vi "Combine axes arrays.vi"(2 "Axes subset 1":string[](array[string]), 3 "Axes subset 2":string[](array[string])) -> (14 "Combined axes":string[](array[string]), 15 "Double axes":string[](array[string]))   [LabVIEW 2020]
doc: "This VI combines axes from Axes subset 1 and Axes subset 2 and returns the combined and sorted axes array plus axes which had double entries."
panel:
  # "This vi combines axes from Axes subset 1 and Axes subset 2 and returns the \ncombined and sorted axes array plus axes which had double entries."
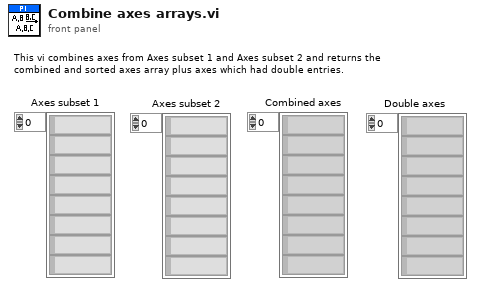
[diagram p1: front panel]
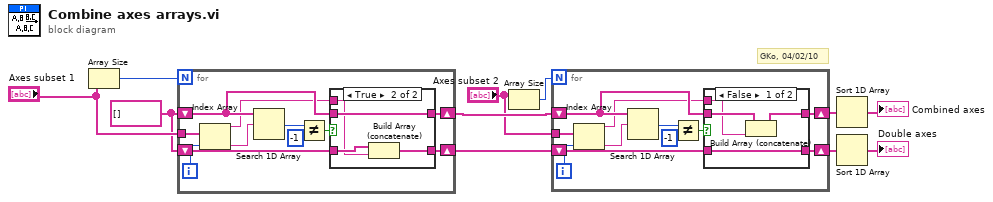
[diagram p0: block diagram]
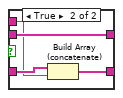
[diagram p2: hidden frame]
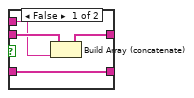
[diagram p3: hidden frame]
diagram:
  w9 = string[] []
  # "GKo, 04/02/10"
  n1 = Array Size(array="Axes subset 1") -> (size(s)=w11:i32)
  n2 = for {
    N: w11 -> [_]
    shift-right: [w20] -> w7
    shift-left: w9 -> [w18]
    tunnel: "Axes subset 1" -> [w19]
    shift-right: [w12] -> w6
    shift-left: w9 -> [w13]
    i -> [w21]
    n3 = Index Array(array=w19, index=w21) -> (element=w17:string)
    n4 = Search 1D Array(1D array=w18, element=w17) -> (index of element=w16:i32)  [unwired: 1 out]
    n5 = Not Equal?(x=w16, y=-1) -> (x != y?=w14:bool)
    n6 = case shown="True" w14 {
      tunnel: [w25 w29] -> w20
      tunnel: w18 -> [w24 w29]
      tunnel: w17 -> [w23 w26]
      tunnel: [w22 w28] -> w12
      tunnel: w13 -> [w22 w27]
      frame False {
        n7 = Build Array (concatenate)(w24, w23) -> (w25:string[])
      }
      frame True {
        n8 = Build Array (concatenate)(w27, w26) -> (w28:string[])
      }
    }
  }
  n9 = Array Size(array="Axes subset 2") -> (size(s)=w8:i32)
  n10 = for {
    N: w8 -> [_]
    shift-right: [w38] -> w4
    shift-left: w7 -> [w36]
    tunnel: "Axes subset 2" -> [w37]
    shift-right: [w30] -> w2
    shift-left: w6 -> [w31]
    i -> [w39]
    n11 = Index Array(array=w37, index=w39) -> (element=w35:string)
    n12 = Search 1D Array(1D array=w36, element=w35) -> (index of element=w34:i32)  [unwired: 1 out]
    n13 = Not Equal?(x=w34, y=-1) -> (x != y?=w32:bool)
    n14 = case shown="False" w32 {
      tunnel: [w43 w47] -> w38
      tunnel: w36 -> [w42 w47]
      tunnel: w35 -> [w41 w44]
      tunnel: [w40 w46] -> w30
      tunnel: w31 -> [w40 w45]
      frame False {
        n15 = Build Array (concatenate)(w42, w41) -> (w43:string[])
      }
      frame True {
        n16 = Build Array (concatenate)(w45, w44) -> (w46:string[])
      }
    }
  }
  n17 = Sort 1D Array(array=w4) -> (sorted array=→"Combined axes":string[])
  n18 = Sort 1D Array(array=w2) -> (sorted array=→"Double axes":string[])
